vi "Configure Source Gamma Correction.vi"(7 "Magnitude Value (0)":dbl, 8 "error in (no error)":errorcluster, 9 "Phase Value (0)":dbl, 10 "Enable SGamma Correction (T: Enable)":bool=TRUE, 11 "VISA resource name":refnum<visa-resource-name>) -> (0 "error out":errorcluster, 3 "VISA resource name out":refnum<visa-resource-name>)   [LabVIEW 2018, in "Agilent U2000 Series.lvlib"]
doc: "Sets the magnitude and phase values of the source reflection coefficient. \n\nNote: \nThis VI is only applicable for U2040 X-Series."
uses:
  Agilent U2000 Series.lvlib
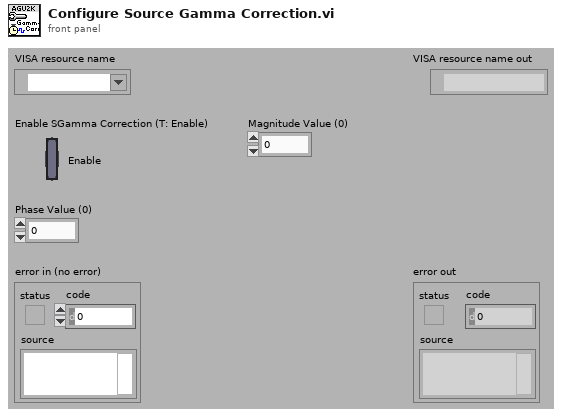
[diagram p1: front panel]
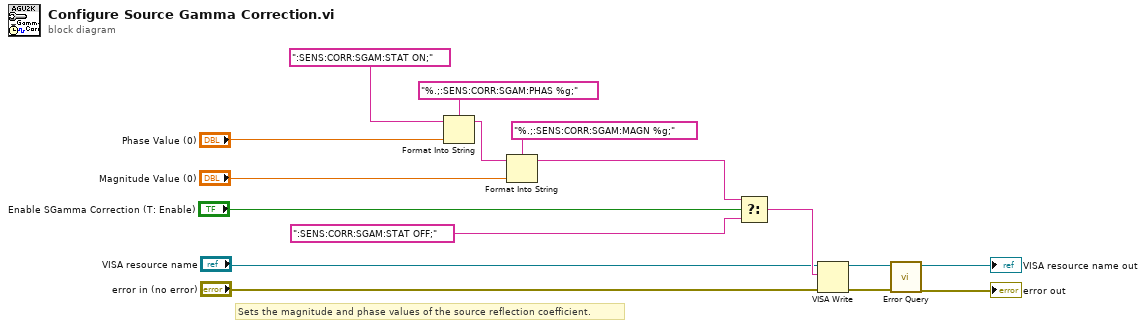
[diagram p0: block diagram]
diagram:
  # "Sets the magnitude and phase values of the source reflection coefficient."
  n1 = Format Into String(format string="%.;:SENS:CORR:SGAM:PHAS %g;", initial string=":SENS:CORR:SGAM:STAT ON;", "Phase Value (0)") -> (resulting string=w6:string)  [unwired: 1 in, 1 out]
  n2 = Format Into String(format string="%.;:SENS:CORR:SGAM:MAGN %g;", initial string=w6, "Magnitude Value (0)") -> (resulting string=w4:string)  [unwired: 1 in, 1 out]
  n3 = Select(t=w4, s="Enable SGamma Correction (T: Enable)", f=":SENS:CORR:SGAM:STAT OFF;") -> (s? t:f=w3:string)
  n4 = VISA Write(VISA resource name="VISA resource name", write buffer=w3, error in (no error)="error in (no error)") -> (VISA resource name out=w16:refnum<visa-resource-name>, error out=w15:errorcluster)  [unwired: 1 out]
  n5 = call "Error Query.vi"("error in (no error)"=w15, "VISA resource name"=w16) -> ("error out"=→"error out":errorcluster, "VISA resource name out"=→"VISA resource name out":refnum<visa-resource-name>)  [unwired: 6 in, 2 out]
